vi "CSM - Argument Token.vi"(5 "Arguments":string) -> (1 "Arg Token":string, 2 "Arguments(dup)":string)   [LabVIEW 2017, in "CSM Shared.lvlib"]
uses:
  CSM Shared.lvlib
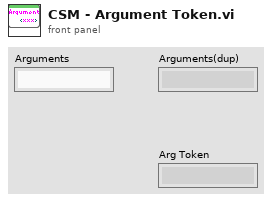
[diagram p1: front panel]
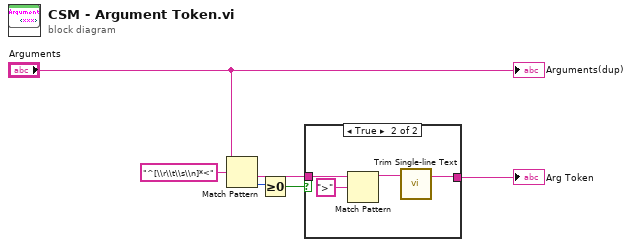
[diagram p0: block diagram]
diagram:
  n1 = Match Pattern(string="Arguments", regular expression="^[\\r\\t\\s\\n]*<") -> (after substring=w3:string, offset past match=w4:i32)  [unwired: 1 in, 2 out]
  n2 = Greater Or Equal To 0?(x=w4) -> (x >= 0?=w5:bool)
  n3 = case shown="True" w5 {
    tunnel: w3 -> [_ w9]
    tunnel: [_ w7] -> w6
    frame False {
    }
    frame True {
      n4 = Match Pattern(string=w9, regular expression=">") -> (before substring=w8:string)  [unwired: 1 in, 3 out]
      n5 = call "Trim Single-line Text.vi"("single-line text"=w8) -> ("trimed text"=w7:string)  [unwired: 2 in]
    }
  }
  "Arg Token" <- w6
  "Arguments(dup)" <- "Arguments"
